vi "2.vi"() -> ()   [LabVIEW 2018]
panel:
  in  "stop":bool
  out "IMC":dbl(slide) scale=10.0..40.0
  in  "?":dbl
  in  "altura":dbl
  in  "peso":dbl
  # "Imdice de masa corporal"
  # "kilogramos"
  # "centimetros"
  # "metro"
  # "obesidad"
  # "sobrepeso"
  # "peso normal"
  # "bajo peso"
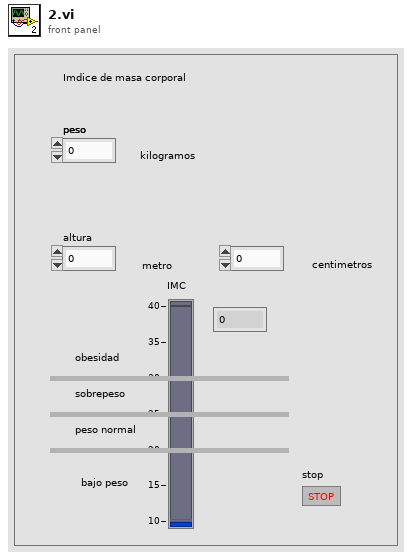
[diagram p1: front panel]
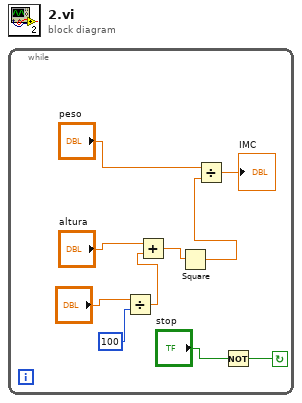
[diagram p0: block diagram]
diagram:
  n1 = while {
    stop <- w10 continue-if-true
    n2 = Divide(x="?", y=100) -> (x/y=w1:dbl)
    n3 = Add(x="altura", y=w1) -> (x+y=w4:dbl)
    n4 = Square(x=w4) -> (x^2=w5:dbl)
    n5 = Divide(x="peso", y=w5) -> (x/y=→"IMC":dbl)
    n6 = Not(x="stop") -> (.not. x?=w10:bool)
  }
